vi "waveformGraph.vi"() -> ()   [LabVIEW 2017]
panel:
  out "Waveform Graph":dbl[][](graph)
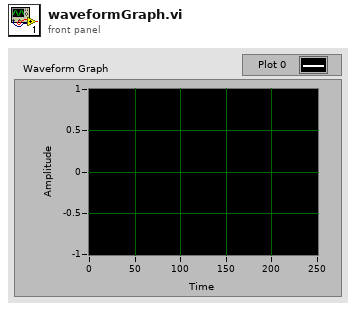
[diagram p1: front panel]
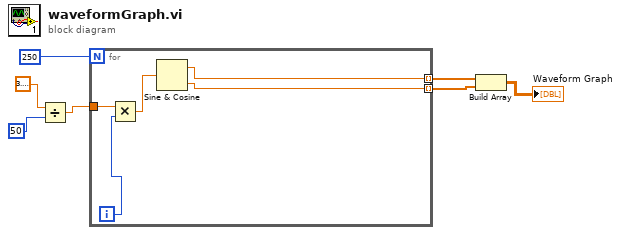
[diagram p0: block diagram]
diagram:
  n1 = Divide(x=3.141592653589793, y=50) -> (x/y=w4:dbl)
  n2 = for {
    N: 250 -> [_]
    tunnel: w4 -> [w11]
    tunnel: [w9] -> w3 mode=indexing
    tunnel: [w8] -> w2 mode=indexing
    i -> [w12]
    n3 = Multiply(x=w11, y=w12) -> (x*y=w10:dbl)
    n4 = Sine & Cosine(0:w10) -> (1:w9:dbl, 2:w8:dbl)
  }
  n5 = Build Array(w3, w2) -> (→"Waveform Graph":dbl[][])
